vi "Datum_Turntable_Image.vi"(3 "Mode":T9=enum."Run VI", 5 "Traverse line In":T6={"Start X"=0.0, "Start Y"=nan, "Start Z"=nan, "End X"=nan, "End Y"=nan, "End Z"=nan, "No. of pts."=0, "Spacing"=enum."N/A", "Filename"=path "C:/Enflo_Data_Local/2016/EnFlo_Tunnel/Paul_Hayden/Calibrations/Cal_03-2016/Datum_Turntable.xls", "Tunnel Speed"=nan, "Averaging time (min)"=nan, "Extra Commands"="", "Carrier_1 Q (l/min)"=nan, "Carrier_2 Q (l/min)"=nan, "Trace Gas Concentration (%)"=nan, "Specific Arguments"="Datum_Turntable_Image.vi ", "Comments"="", "Row No"=0, "Row Type Selector"=enum."Run VI Named:", "Completion time"="12:59  18-03-2016", "Row Duration (mins)"=0.08333333333333333, "No. of Valid pts."=0, "Meas Setup File"="Trav_Cam_Picture.xls"} {"Carrier_2 Q (l/min)" format="%#.2f"; "Row Duration (mins)" format="%#.1f"; "Row No" min=0; "Trace Gas Concentration (%)" min=0.0 format="%#_4f"; "Carrier_1 Q (l/min)" format="%#.2f"; "Tunnel Speed" format="%#.2f"; "Start X" format="%#.2f"; "Start Y" format="%#.2f"; "Start Z" format="%#.2f"; "End X" format="%#.2f"; "End Y" format="%#.2f"; "End Z" format="%#.2f"; "Averaging time (min)" min=0.0 format="%#.2f"}) -> (0 "Error Message":string, 1 "Status":T5, 2 "Traverse line Out":T6={"Start X"=0.0, "Start Y"=nan, "Start Z"=nan, "End X"=nan, "End Y"=nan, "End Z"=nan, "No. of pts."=0, "Spacing"=enum."N/A", "Filename"=path "C:/Enflo_Data_Local/2016/EnFlo_Tunnel/Paul_Hayden/Calibrations/Cal_03-2016/Datum_Turntable.xls", "Tunnel Speed"=nan, "Averaging time (min)"=nan, "Extra Commands"="", "Carrier_1 Q (l/min)"=nan, "Carrier_2 Q (l/min)"=nan, "Trace Gas Concentration (%)"=nan, "Specific Arguments"="Datum_Turntable_Image.vi ", "Comments"="", "Row No"=0, "Row Type Selector"=enum."Run VI Named:", "Completion time"="12:59  18-03-2016", "Row Duration (mins)"=0.08333333333333333, "No. of Valid pts."=0, "Meas Setup File"="Trav_Cam_Picture.xls"} {"Carrier_2 Q (l/min)" format="%#.2f"; "Row Duration (mins)" format="%#.1f"; "Row No" min=0; "Trace Gas Concentration (%)" min=0.0 format="%#_4f"; "Carrier_1 Q (l/min)" format="%#.2f"; "Tunnel Speed" format="%#.2f"; "Start X" format="%#.2f"; "Start Y" format="%#.2f"; "Start Z" format="%#.2f"; "End X" format="%#.2f"; "End Y" format="%#.2f"; "End Z" format="%#.2f"; "Averaging time (min)" min=0.0 format="%#.2f"})   [LabVIEW 2015]
uses:
  Gen Trav/Traverse_cluster.ctl
  Gen Trav/Spacing.ctl
  Controls/Multi_run_mode.ctl
  Controls/User_Specific_mode.ctl
  Gen Trav/Multi_Run_Status.ctl
  Utilities/Image acquisition and processing/Feature detection/Typedefs/ROI bounds.ctl
  Utilities/Image acquisition and processing/Feature detection/Typedefs/Theta range.ctl
  Camera Server/Camera enum/Camera enum.ctl
  Utilities/Image acquisition and processing/Feature detection/Typedefs/Top level controls.ctl
  Gen Trav/Trav_mode.ctl
  Utilities/Image acquisition and processing/Feature detection/Typedefs/Txy range.ctl
panel:
  out "Deg for Relaxing Drive":dbl
  in  "Controls":T1={"Auto ROI (for rot.)"=TRUE, "Apply scaling"=FALSE, "Apply rotation"=TRUE, "Apply Tx"=TRUE, "Apply Ty"=TRUE, "Keep proc. img"=FALSE}
  in  "Quality":u32=750 max=1000
  in  "Camera":T2="TurntableCam"
  in  "Theta range (deg)":T3={"theta max (deg)"=180.0, "theta min (deg)"=-180.0}
  in  "ROI to crop (pixels)":T4={"Xmax"=1612, "Ymax"=1300, "Xmin"=660, "Ymin"=226}
  # "X           Y            Z"
  # "Start"
  # "End"
  # "X           Y            Z"
  # "Start"
  # "End"
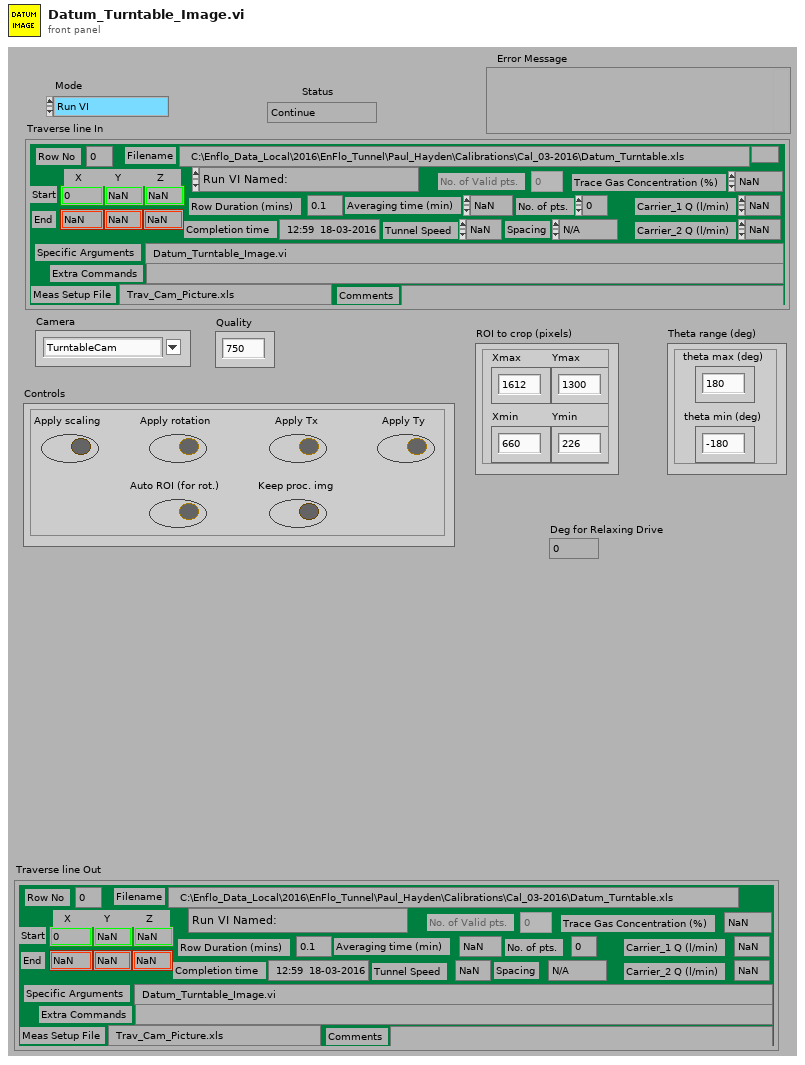
[diagram p1: front panel]
types:
  T1 = typedef "Top level controls.ctl" = cluster{"Auto ROI (for rot.)":bool, "Apply scaling":bool, "Apply rotation":bool, "Apply Tx":bool, "Apply Ty":bool, "Keep proc. img":bool}
  T2 = typedef "Camera enum.ctl" = string
  T3 = typedef "Theta range.ctl" = cluster{"theta max (deg)":dbl, "theta min (deg)":dbl}
  T4 = typedef "ROI bounds.ctl" = cluster{"Xmax":i32, "Ymax":i32, "Xmin":i32, "Ymin":i32}
  T5 = typedef "Multi_Run_Status.ctl" = enum16{"Continue", "Jump to Next Point", "Jump to Next Row", "Jump To Fall Back", "Terminate Run"}
  T6 = typedef "Traverse_cluster.ctl" = cluster{"Start X":sgl, "Start Y":sgl, "Start Z":sgl, "End X":sgl, "End Y":sgl, "End Z":sgl, "No. of pts.":i32, "Spacing":T7, "Filename":path, "Tunnel Speed":dbl, "Averaging time (min)":dbl, "Extra Commands":string, "Carrier_1 Q (l/min)":dbl, "Carrier_2 Q (l/min)":dbl, "Trace Gas Concentration (%)":dbl, "Specific Arguments":string, "Comments":string, "Row No":i32, "Row Type Selector":T8, "Completion time":string, "Row Duration (mins)":dbl, "No. of Valid pts.":i32, "Meas Setup File":string}
  T7 = typedef "Spacing.ctl" = enum16{"Linear", "Log", "Gauss", "Specified", "N/A"}
  T8 = typedef "Multi_run_mode.ctl" = enum16{"Move Traverse Only", "Set Tunnel Speed Only", "Set Source Only", "Set Measurement Conditions", "Single Measurement", "Vertical Profile", "Lateral Profile", "Longitudinal Profile", "Explore Volume", "Multi-Axis Profile", "Auto Calibrate", "Meas Fast FID Bkgnd", "Check Beam Power", "Scanning Valve Measurement", "Run VI Named:", "Set ADAM Ch", "Wait (minutes)", "Send Message", "Synchronize With:", "Fall Back to this Row", "Turn Off Row Repeating", "Blank Row", "Traverse 3D Volume"}
  T9 = typedef "User_Specific_mode.ctl" = enum16{"Check VI only", "Run VI"}
  T10 = typedef "Trav_mode.ctl" = enum16{"Move traverse", "Read traverse position", "Teach Position"}
  T11 = typedef "Txy range.ctl" = cluster{"Tx max (pix)":i32, "Tx min (pix)":i32, "Ty max (pix)":i32, "Ty min (pix)":i32}
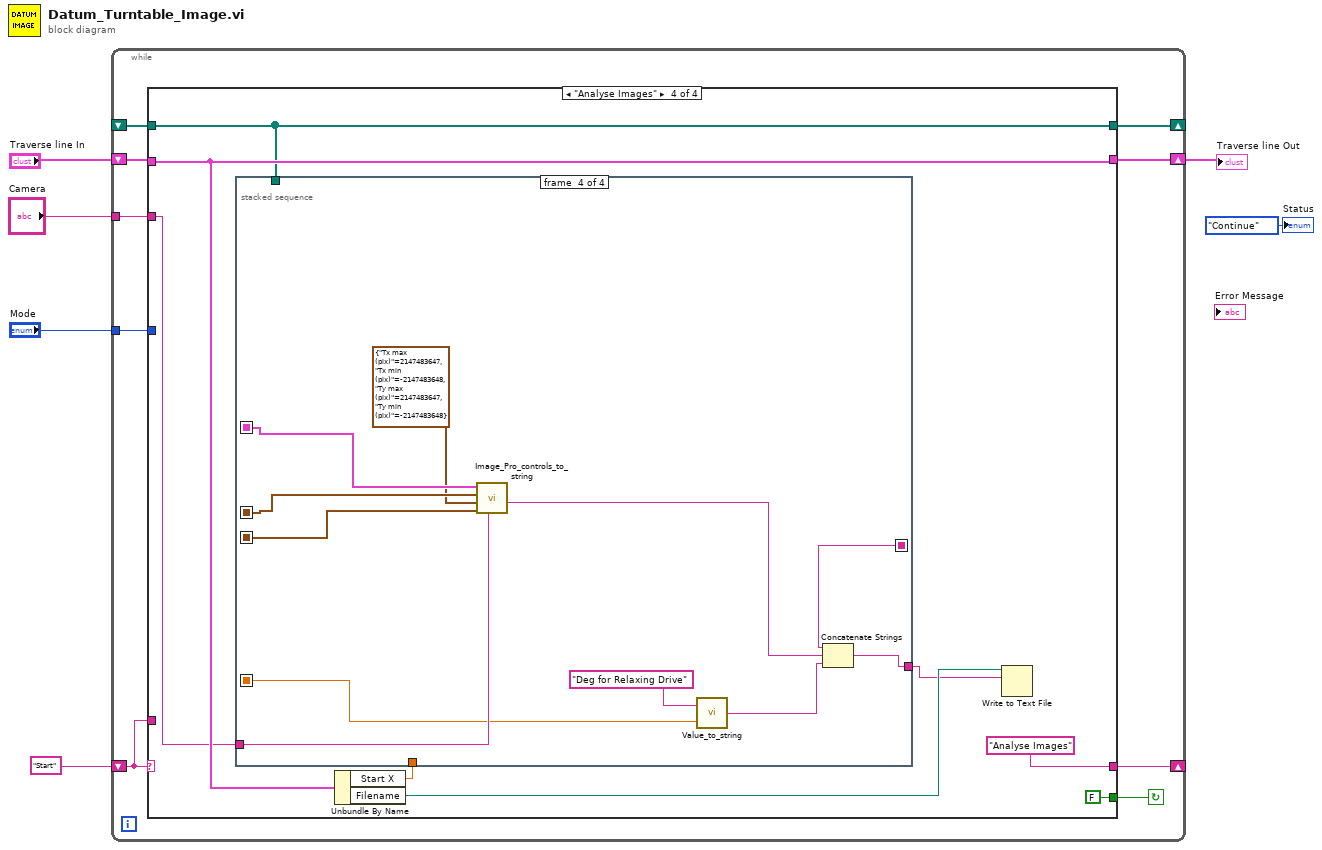
[diagram p0: block diagram]
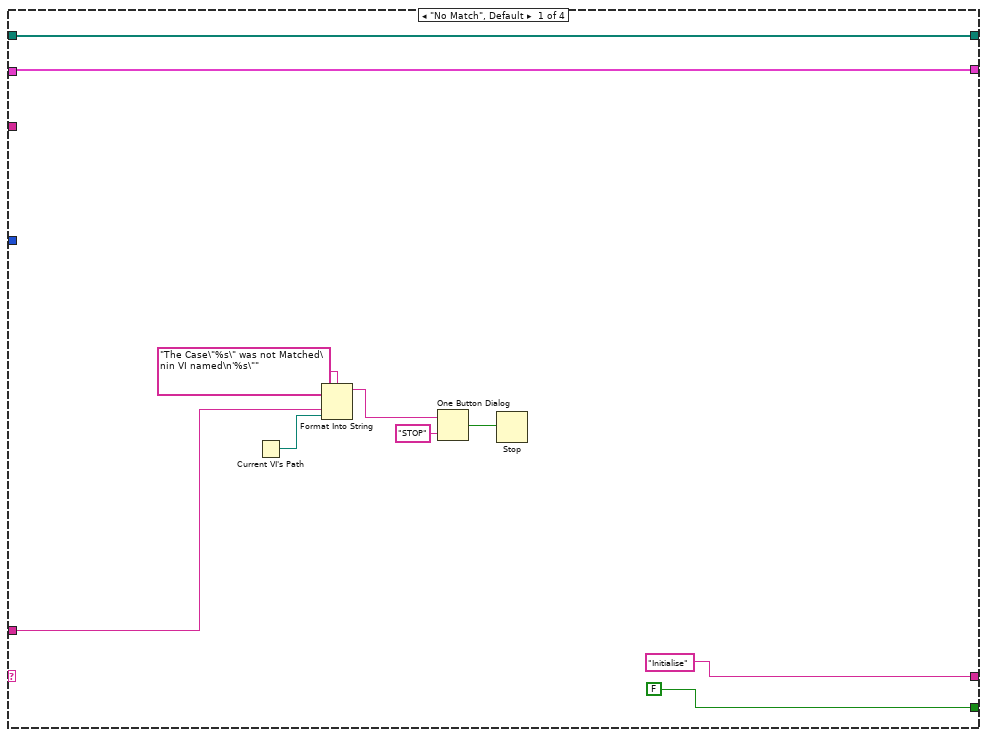
[diagram p2: hidden frame]
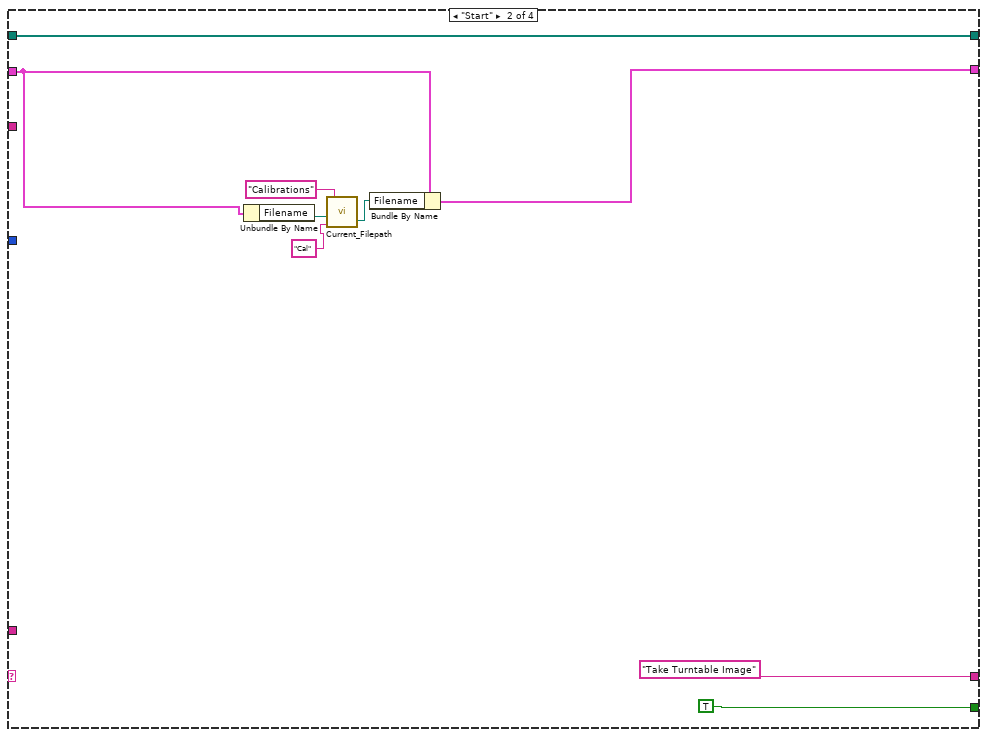
[diagram p3: hidden frame]
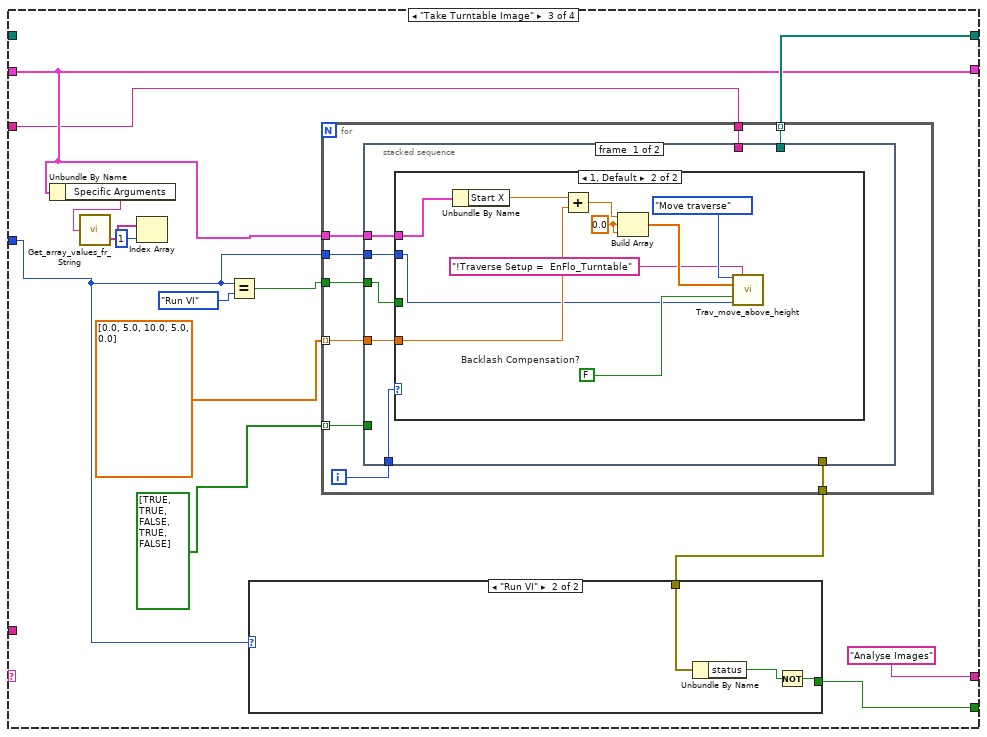
[diagram p4: hidden frame]
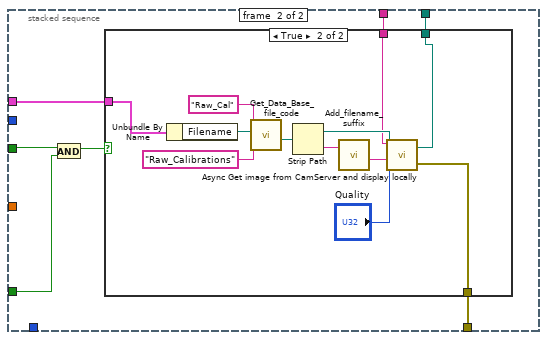
[diagram p6: hidden frame]
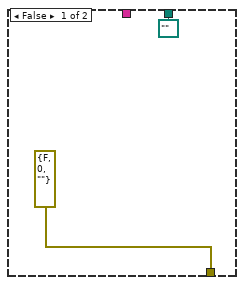
[diagram p7: hidden frame]
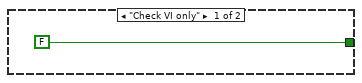
[diagram p8: hidden frame]
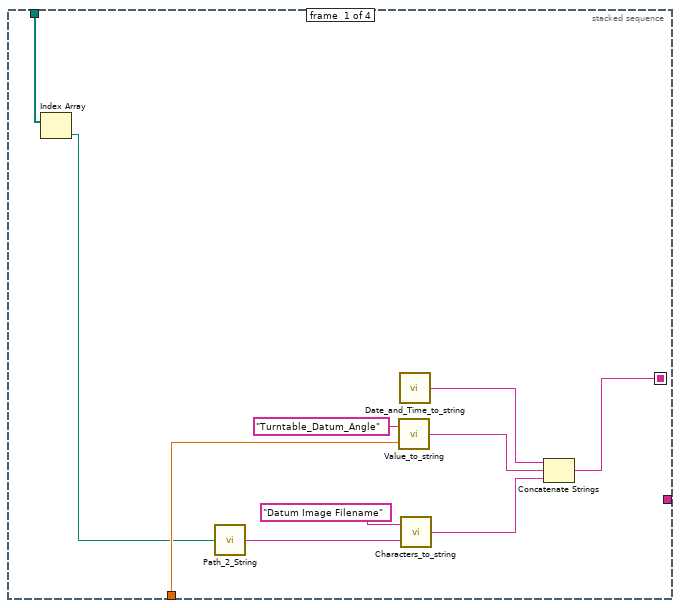
[diagram p9: hidden frame]
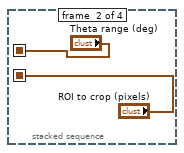
[diagram p10: hidden frame]
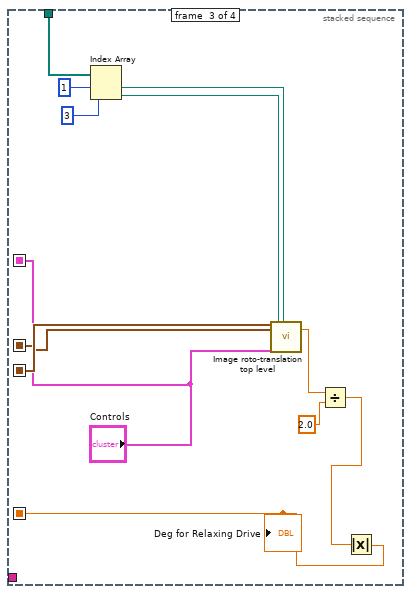
[diagram p11: hidden frame]
diagram:
  n1 = while {
    shift-left: "Start" -> [w13]
    shift-right: [w14] -> _
    tunnel: "Mode" -> [w12]
    shift-right: [w10] -> w2
    shift-left: "Traverse line In" -> [w11]
    shift-right: [w9] -> _
    shift-left: _ -> [w8]
    tunnel: "Camera" -> [w7]
    stop <- w15 continue-if-true
    n2 = case shown="\"Analyse Images\"" w13 {
      tunnel: [FALSE TRUE w46 FALSE] -> w15
      tunnel: ["Initialise" "Take Turntable Image" "Analyse Images" "Analyse Images"] -> w14
      tunnel: w13 -> [w20 _ _ _]
      tunnel: w12 -> [_ _ w35 _]
      tunnel: w11 -> [w17 w29 w44 w103]
      tunnel: [w17 w28 w44 w103] -> w10
      tunnel: [w16 w27 w47 w98] -> w9
      tunnel: w8 -> [w16 w27 _ w98]
      tunnel: w7 -> [_ _ w40 w100]
      frame "No Match", Default {
        n3 = Current VI's Path() -> (path=w19:path)
        n4 = Format Into String(format string="The Case\"%s\" was not Matched\nin VI named\n'%s\"" ("Format String"), w20, w19) -> (resulting string=w23:string)  [unwired: 2 in, 1 out]
        n5 = One Button Dialog(message=w23, button name ("OK")="STOP") -> (true=w21:bool)
        n6 = Stop(stop? (T)=w21) -> ()
      }
      frame "Start" {
        n7 = Unbundle By Name(w29) -> ("Filename"=w31:path)
        n8 = call "Current_Filepath.vi"("Short_Name"="Cal" ("Data Type"), "Filename in"=w31, "Data Type"="Calibrations") -> ("Filename Out"=w26:path)  [unwired: 1 in, 1 out]
        n9 = Bundle By Name(cluster=w29, "Filename"=w26) -> (w28:T6)
      }
      frame "Take Turntable Image" {
        n10 = Unbundle By Name(w44) -> ("Specific Arguments"=w43:string)
        n11 = call "Get_array_values_fr_String.vi"("String Value"=w43) -> ("String array"=w42:string[])  [unwired: 1 out]
        n12 = Index Array(array=w42, index=1) -> ()  [unwired: 1 out]
        n13 = Equal?(x=w35, y=User_Specific_mode."Run VI" ("Mode")) -> (x = y?=w37:bool)
        n14 = for {
          tunnel: [w57] -> w47 mode=indexing
          tunnel: w37 -> [w56]
          tunnel: [w55] -> w45
          tunnel: w44 -> [w54]
          tunnel: w40 -> [w53]
          tunnel: sgl[] [0.0, 5.0, 10.0, 5.0, 0.0] ("Array") -> [w52] mode=indexing
          tunnel: bool[] [TRUE, TRUE, FALSE, TRUE, FALSE] ("Array") -> [w50] mode=indexing
          tunnel: w35 -> [w49]
          i -> [w51]
          n15 = stacked-sequence {
            tunnel: [_ w79] -> w57
            tunnel: w56 -> [w59 w75]
            tunnel: [_ w78] -> w55
            tunnel: w54 -> [w62 w77]
            tunnel: w53 -> [_ w76]
            tunnel: w52 -> [w61 _]
            tunnel: w51 -> [w60 _]
            tunnel: w50 -> [_ w73]
            tunnel: w49 -> [w58 _]
            frame #0 {
              n16 = case shown="1, Default" w60 {
                tunnel: w62 -> [_ w72]
                tunnel: w61 -> [_ w71]
                tunnel: w59 -> [_ _]
                tunnel: w58 -> [_ w64]
                frame 0 {
                }
                frame 1, Default {
                  w65 = FALSE  # Backlash Compensation?
                  w68 = sgl 0.0 ("element")
                  n17 = Unbundle By Name(w72) -> ("Start X"=w70:sgl)
                  n18 = Add(x=w70, y=w71) -> (x+y=w69:sgl)
                  n19 = Build Array(w69, w68, w68) -> (w67:sgl[])
                  n20 = call "Trav_move_above_height.vi"("Mode"=Trav_mode."Move traverse", "Extra Command String"="!Traverse Setup =  EnFlo_Turntable", "New Position"=w67, "Backlash Compensation?"=w65, "Simulate/Run"=w64) -> ()  [unwired: 8 in, 3 out]
                }
              }
            }
            frame #1 {
              n21 = And(x=w75, y=w73) -> (x .and. y?=w74:bool)
              n22 = case shown="True" w74 {
                tunnel: w77 -> [_ w91]
                tunnel: [path "" ("stripped path") w84] -> w79
                tunnel: [errorcluster {"status"=FALSE, "code"=0, "source"=""} ("Error Out") w86] -> w78
                tunnel: w76 -> [_ w82]
                frame False {
                }
                frame True {
                  n23 = Unbundle By Name(w91) -> ("Filename"=w88:path)
                  n24 = call "Get_Data_Base_file_code.vi"("Data Type"="Raw_Calibrations", "Results Filename"=w88, "Short_Name"="Raw_Cal" ("Data Type")) -> ("Raw Data File Name"=w85:path)  [unwired: 1 in, 3 out]
                  n25 = Strip Path(path=w85) -> (stripped path=w87:path, name=w90:string)
                  n26 = call "Add_filename_suffix.vi"("Filename"=w90) -> ("Base name"=w89:string)  [unwired: 1 in, 3 out]
                  n27 = call "Async Get image from CamServer and display locally.vi"("Quality"="Quality", "Image name"=w89, "Image directory path"=w87, "Camera"=w82) -> ("Error out"=w86:errorcluster, "Image file path"=w84:path)
                }
              }
            }
          }
        }
        n28 = case shown="\"Run VI\"" w35 {
          tunnel: [FALSE w96] -> w46
          tunnel: w45 -> [_ w97]
          frame "Check VI only" {
          }
          frame "Run VI" {
            n29 = Unbundle By Name(w97) -> ("status"=w95:bool)
            n30 = Not(x=w95) -> (.not. x?=w96:bool)
          }
        }
      }
      frame "Analyse Images" {
        n31 = Unbundle By Name(w103) -> ("Start X"=w99:sgl, "Filename"=w102:path)
        n32 = stacked-sequence {
          seq-local: [w110 _ _ _] -> [_ _ _ w133]
          seq-local: [_ "Theta range (deg)" _ _] -> [_ _ w123 w138]
          seq-local: [_ "ROI to crop (pixels)" _ _] -> [_ _ w124 w137]
          seq-local: [_ _ "Controls" _] -> [_ _ _ w139]
          seq-local: [_ _ w118 _] -> [_ _ _ w134]
          tunnel: [_ _ _ w130] -> w101
          tunnel: w100 -> [_ _ _ w140]
          tunnel: w99 -> [w108 _ _ _]
          tunnel: w98 -> [w107 _ w129 _]
          frame #0 {
            n33 = Index Array(array=w107) -> (element=w106:path)  [unwired: 1 in]
            n34 = call "Path_2_String.vi"("Real Path"=w106) -> ("Path String"=w114:string)
            n35 = call "Value_to_string.vi"("Value"=w108, "Label for value"="Turntable_Datum_Angle") -> ("Output string"=w112:string)  [unwired: 1 in]
            n36 = call "Date_and_Time_to_string.vi"() -> ("Date and time (spreadsheet)"=w111:string)
            n37 = call "Characters_to_string.vi"("Characters to write"=w114, "Label for characters"="Datum Image Filename") -> ("Output string"=w109:string)
            n38 = Concatenate Strings(w111, w112, w109) -> (w110:string)
          }
          frame #1 {
          }
          frame #2 {
            n39 = Index Array(array=w129, index #1=1 ("index"), index #2=3 ("index")) -> (element #1=w125:path, element #2=w126:path)
            n40 = call "Image roto-translation top level.vi"("ROI to crop (pixels)"=w124, "Theta range (deg)"=w123, "Controls"="Controls", "Test image file path"=w126, "Reference image file path"=w125) -> ("Rotation (deg)"=w122:dbl)  [unwired: 8 in, 6 out]
            n41 = Divide(x=w122, y=2.0) -> (x/y=w120:dbl)
            n42 = Absolute Value(x=w120) -> (abs(x)=w118:dbl)
            "Deg for Relaxing Drive" <- w118
          }
          frame #3 {
            n43 = call "Image_Pro_controls_to_string.vi"("Camera"=w140, "ROI to crop (pixels)"=w137, "Txy range (pixels)"=T11 {"Tx max (pix)"=2147483647, "Tx min (pix)"=-2147483648, "Ty max (pix)"=2147483647, "Ty min (pix)"=-2147483648}, "Theta range (deg)"=w138, "Controls"=w139) -> ("Setup String"=w132:string)  [unwired: 6 in]
            n44 = call "Value_to_string.vi"("Value"=w134, "Label for value"="Deg for Relaxing Drive" ("Label for characters")) -> ("Output string"=w131:string)  [unwired: 1 in]
            n45 = Concatenate Strings(w133, w132, w131) -> (w130:string)
          }
        }
        n46 = Write to Text File(file (use dialog)=w102, text=w101) -> ()  [unwired: 2 in, 3 out]
      }
    }
  }
  "Traverse line Out" <- w2
  "Status" <- Multi_Run_Status."Continue" ("Status")
